vi "ActionVIOnLoad.vi"(8 "error in (no error)":errorcluster, 11 "Device Item Ref in":T1 format="%.0x") -> (0 "error out":errorcluster, 3 "Device Item Ref out":T1 format="%.0x")   [LabVIEW 2020, in "AIM ARINC 664 System Explorer.lvlib" / "Implementation.lvlib"]
uses:
  Implementation.lvlib
  <vilib>/NI VeriStand/Custom Device API/Custom Device Item Ref.ctl
  NationalInstruments.VeriStand.SystemDefinitionAPI
  <vilib>/NI VeriStand/Custom Device API/Custom Device API.lvlib
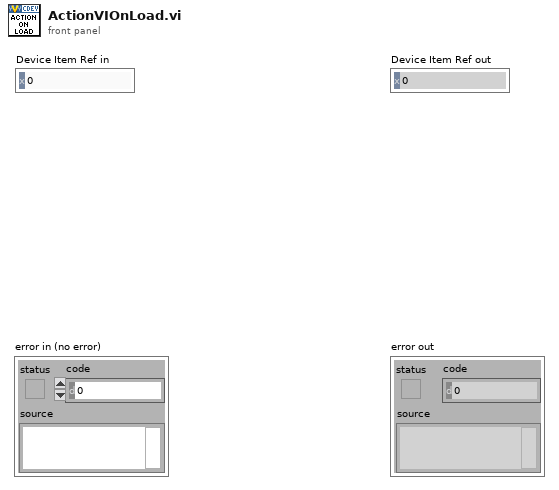
[diagram p1: front panel]
types:
  T1 = typedef "Custom Device API.lvlib/Custom Device Item Ref.ctl" = u64
  T2 = typedef "Custom Device API.lvlib/Custom Device Item Info.ctl" = cluster{"Name":string, "Is Channel":bool, "GUID":string, "Is Waveform":bool}
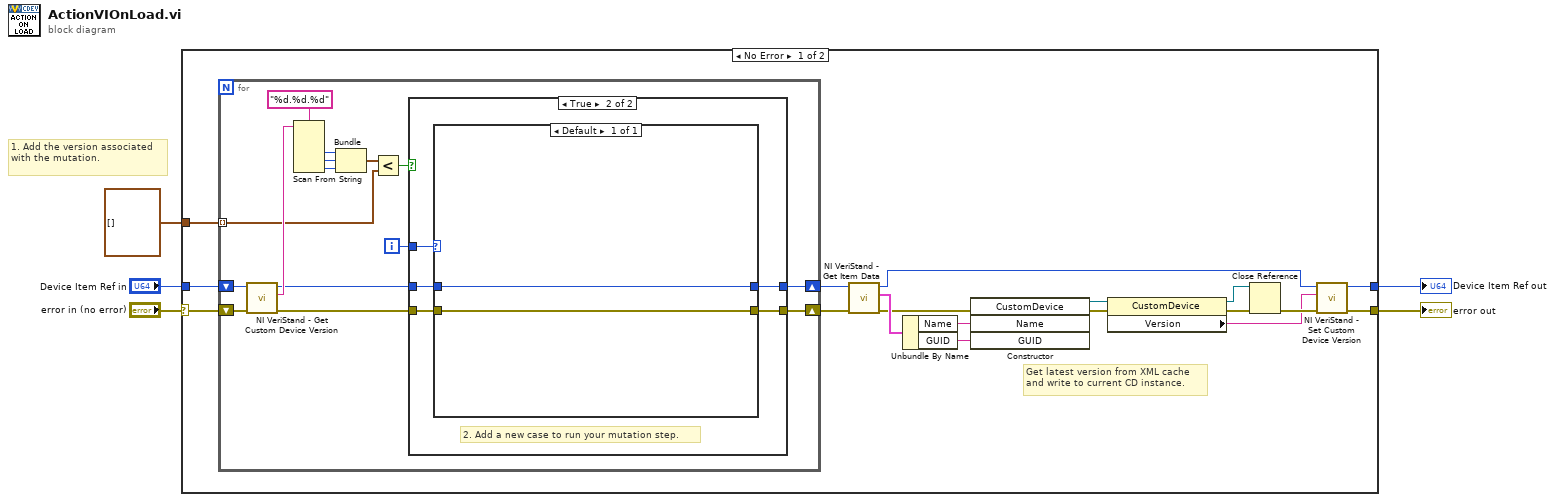
[diagram p0: block diagram]
diagram:
  # "1. Add the version associated with the mutation."
  n1 = case shown="No Error" "error in (no error)" {
    selector: "error in (no error)" -> [w23 w49]
    tunnel: [w6 w49] -> w3
    tunnel: "Device Item Ref in" -> [w22 w48]
    tunnel: [w7 w48] -> w2
    tunnel: cluster{i32, i32, i32}[] [] -> [w21 _]
    frame No Error {
      # "Get latest version from XML cache\nand write to current CD instance."
      n2 = for {
        shift-right: [w29] -> w19
        shift-left: w23 -> [w34]
        shift-right: [w27] -> w20
        shift-left: w22 -> [w33]
        tunnel: w21 -> [w24] mode=indexing
        i -> [w26]
        n3 = call <vilib>:"NI VeriStand - Get Custom Device Version.vi"("error in (no error)"=w34, "Device Ref in"=w33) -> ("error out"=w30:errorcluster, "Value"=w32:string, "Device Ref out"=w28:T1)  [unwired: 7 in]
        n4 = Scan From String(format string="%d.%d.%d", input string=w32) -> (output 1=w36:i32, output 2=w37:i32, output 3=w25:i32)  [unwired: 5 in, 3 out]
        n5 = Bundle(w36, w37, w25) -> (w38:cluster{i32, i32, i32})  [unwired: 1 in]
        n6 = Less?(x=w38, y=w24) -> (x < y?=w31:bool)
        n7 = case shown="True" w31 {
          tunnel: w30 -> [w40 w45]
          tunnel: [w40 w44] -> w29
          tunnel: w28 -> [w39 w41]
          tunnel: [w39 w42] -> w27
          tunnel: w26 -> [_ w43]
          frame False {
          }
          frame True {
            # "2. Add a new case to run your mutation step."
            n8 = case shown="Default" w43 {
              tunnel: w45 -> [w47]
              tunnel: [w47] -> w44
              tunnel: [w46] -> w42
              tunnel: w41 -> [w46]
              frame Default {
              }
            }
          }
        }
      }
      n9 = call <vilib>:"NI VeriStand - Get Item Data.vi"("error in (no error)"=w19, "Item Ref in"=w20) -> ("error out"=w15:errorcluster, "Item Info"=w18:T2, "Item Ref out"=w8:T1)  [unwired: 6 in, 1 out]
      n10 = Unbundle By Name(w18) -> ("Name"=w17:string, "GUID"=w16:string)
      n11 = constructor class="CustomDevice"(error in=w15, "Name"=w17, "GUID"=w16) -> (reference out=w14:refnum<k24>, error out=w13:errorcluster)  [unwired: 2 in, 3 out]
      n12 = property class="CustomDevice"(reference=w14, error in=w13) -> (reference out=w11:refnum<k24>, error out=w12:errorcluster, "Version"=w9:string)
      n13 = Close Reference(reference=w11, error in (no error)=w12) -> (error out=w10:errorcluster)
      n14 = call <vilib>:"NI VeriStand - Set Custom Device Version.vi"("error in (no error)"=w10, "Value"=w9, "Device Ref in"=w8) -> ("error out"=w6:errorcluster, "Device Ref out"=w7:T1)  [unwired: 7 in]
    }
    frame Error {
    }
  }
  "error out" <- w3
  "Device Item Ref out" <- w2
